vi "Normalize Vector.vi"(5 "Vector":dbl[](array[numeric]) format="%0.2f") -> (0 "error":i32, 1 "mean":dbl format="%0.2f", 2 "standard deviation":dbl format="%0.2f", 3 "Normalized Vector":dbl[](array[numeric]) format="%0.2f")   [LabVIEW 2020, in "NI_AALBase.lvlib"]
doc: "Normalizes the input vector or matrix using its statistical profile (micro,s), where micro is the <B>mean</B> and s is the <B>standard deviation</B>, to obtain a <B>Normalized Vector</B> or <B>Normalized Matrix</B> whose statistical profile is (0,1)."
uses:
  NI_AALBase.lvlib
  <resource>/lvanlys.dll
panel:
  # "Normalize Vector"
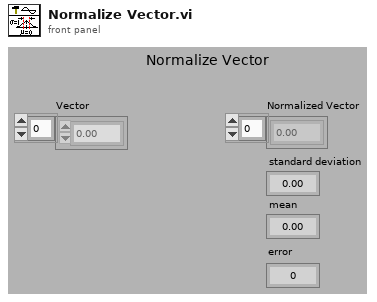
[diagram p1: front panel]
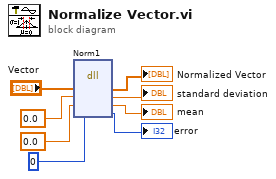
[diagram p0: block diagram]
diagram:
  n1 = dll-call lib="C:/Program Files (x86)/National Instruments/LabVIEW 2020/resource/lvanlys.*" fn="Norm1"("Vector"="Vector", 0.0, 0.0, 0) -> ("Vector"=→"Normalized Vector":dbl[], →"standard deviation":dbl, →"mean":dbl, →"error":i32)  [unwired: 4 in, 2 out]
